vi "DAQinput.vi"() -> ()   [LabVIEW 2018]
panel:
  in  "滑动杆":dbl(slide) scale=100.0..1000.0
  in  "停止":bool
  out "波形图":dynamicdata(graph)
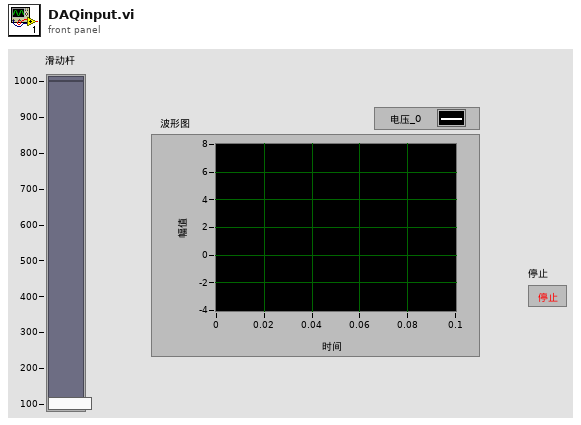
[diagram p1: front panel]
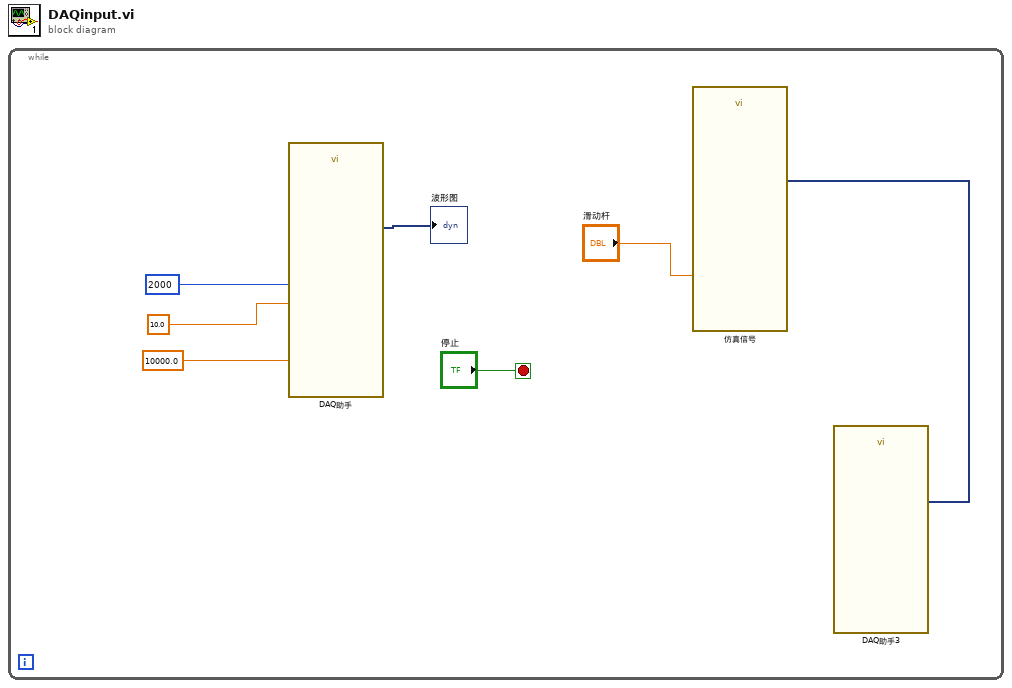
[diagram p0: block diagram]
diagram:
  n1 = while {
    stop <- "停止" stop-if-true
    n2 = call "DAQ助手"("速率"=10000.0, "采样数"=2000, "timeout (s)"=10.0) -> ("data"=→"波形图":dynamicdata)  [unwired: 14 in, 2 out]
    n3 = call "仿真信号"("Frequency"="滑动杆") -> ("方波"=w2:dynamicdata)  [unwired: 13 in, 1 out]
    n4 = call "DAQ助手3"("data"=w2) -> ()  [unwired: 17 in, 2 out]
  }
